vi "Set_DAQmx.vi"(8 "error in (no error)":errorcluster, 11 "Control-Server in":refnum<class "Control-Server.lvclass">) -> (0 "error out":errorcluster, 3 "Control-Server out":refnum<class "Control-Server.lvclass">)   [LabVIEW 2019, in "Control-Server.lvclass"]
uses:
  Control-Server.lvclass
  Config/config_names_def.ctl
  Message/Message.lvclass
  dependecies/ControlsVIs/Clusters-def/Message types.ctl
  Control-Server.lvclass/Control-Server.ctl
  Message/Message.lvclass/Message.ctl
  DAQmxTasks/DAQmxTaskContainer_Emulate/DAQmxTaksContainer_Emulate.lvclass
  C:/Users/elysium/Documents/dev/TRANCON/Classes/DAQmxTasks/DAQmxTaskContainer_General/DAQmxTaksContainer_General.lvclass
  DAQmxTasks/DAQmxTaskContainer/DAQmxTaskContainer.lvclass
  GeneralFunctionality/GeneralFunctionality.lvclass/GeneralFunctionality.ctl
  DAQmxTasks/DAQmxTaskContainer_General/DAQmxTaksContainer_General.lvclass/DAQmxTaksContainer_General.ctl
  Oscilloscope/Oscilloscope.lvclass
  C:/Users/elysium/Documents/dev/TRANCON/Classes/GeneralFunctionality/GeneralFunctionality.lvclass
  Detector/Detector.lvclass
  DAQmxTasks/DAQmxTaskContainer_General/DAQmxTaksContainer_General.lvclass
  Config/Config.lvclass
  GeneralFunctionality/GeneralFunctionality.lvclass
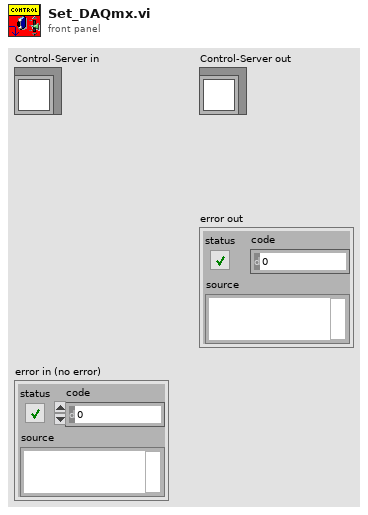
[diagram p1: front panel]
types:
  T1 = typedef "Config.lvclass/config_names_def.ctl" = string
  T2 = typedef "Message types.ctl" = string
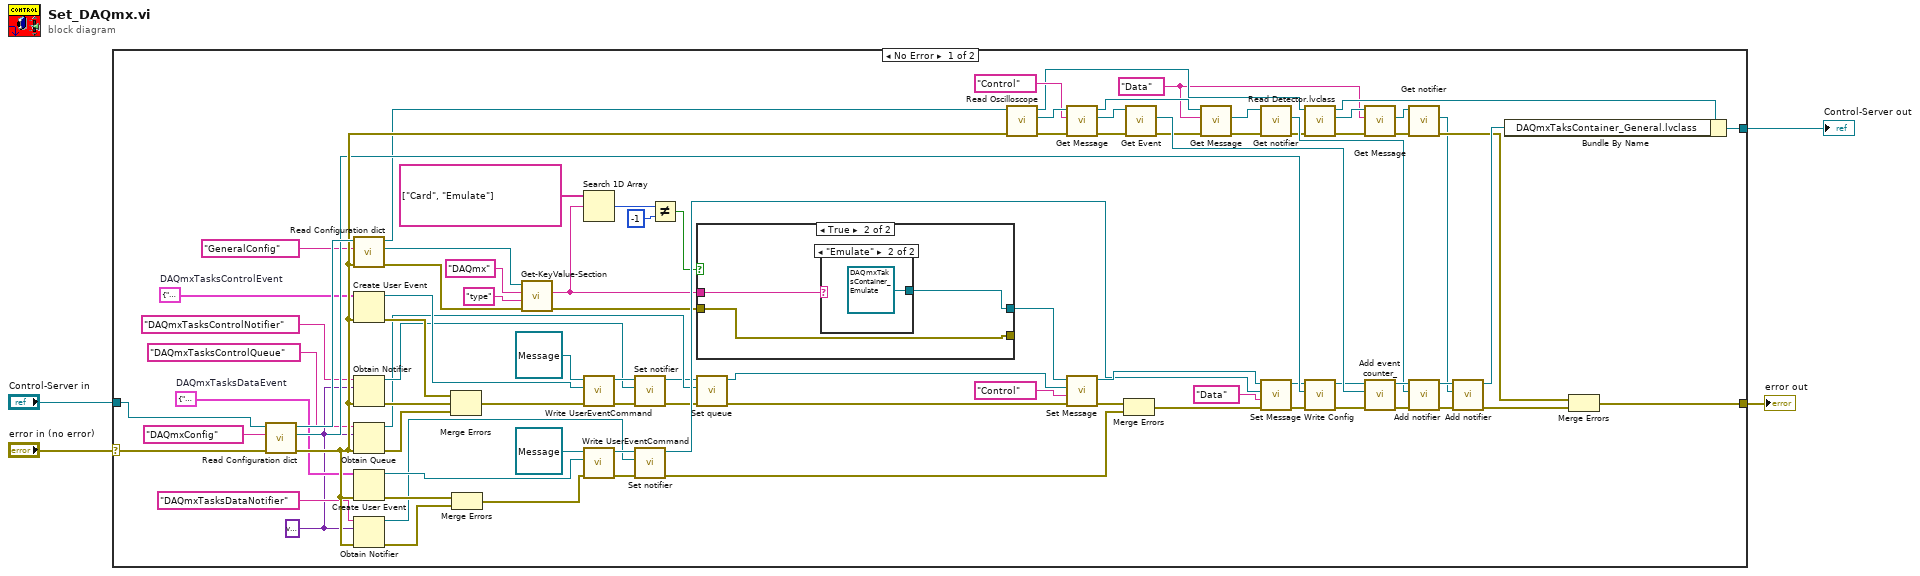
[diagram p0: block diagram]
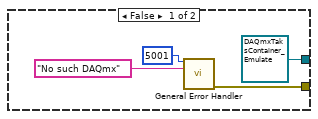
[diagram p2: hidden frame]
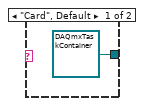
[diagram p3: hidden frame]
diagram:
  n1 = case shown="No Error" "error in (no error)" {
    selector: "error in (no error)" -> [w6 w102]
    tunnel: [w90 w102] -> w4
    tunnel: [w89 w101] -> w3
    tunnel: "Control-Server in" -> [w88 w101]
    frame No Error {
      w24 = T2 "Data" ("Message type")
      w39 = variant
      w71 = cluster{"command":string, "data":variant} {"command"="", "data"=variant}  # DAQmxTasksDataEvent
      w78 = cluster{"command":string, "data":variant} {"command"="", "data"=variant}  # DAQmxTasksControlEvent
      n2 = call "Read Configuration dict.vi"("error in (no error)"=w6, "Config Name"=T1 "DAQmxConfig", "Control in"=w88) -> ("error out"=w85:errorcluster, "Config"=w84:refnum<class "Config.lvclass">, "Control out"=w87:refnum<class "Control-Server.lvclass">)  [unwired: 6 in]
      n3 = call "Read Configuration dict.vi"("error in (no error)"=w85, "Config Name"=T1 "GeneralConfig", "Control in"=w87) -> ("error out"=w19:errorcluster, "Config"=w18:refnum<class "Config.lvclass">, "Control out"=w8:refnum<class "Control-Server.lvclass">)  [unwired: 6 in]
      n4 = Create User Event(user event datatype=w78, error in=w85) -> (user event=w80:refnum<user-event>, error out=w76:errorcluster)
      n5 = Obtain Notifier(name (unnamed)="DAQmxTasksControlNotifier" ("nom (aucun)"), notification data type=w39, error in (no error)=w85) -> (notifier out=w74:refnum<notifier>, error out=w75:errorcluster)  [unwired: 1 in, 1 out]
      n6 = Obtain Queue(name (unnamed)="DAQmxTasksControlQueue", element data type=w39, error in (no error)=w85) -> (queue out=w52:refnum<queue>, error out=w51:errorcluster)  [unwired: 2 in, 1 out]
      n7 = Create User Event(user event datatype=w71, error in=w85) -> (user event=w68:refnum<user-event>, error out=w60:errorcluster)
      n8 = Obtain Notifier(name (unnamed)="DAQmxTasksDataNotifier" ("nom (aucun)"), notification data type=w39, error in (no error)=w85) -> (notifier out=w58:refnum<notifier>, error out=w59:errorcluster)  [unwired: 1 in, 1 out]
      n9 = Merge Errors(w76, w75, w51) -> (w73:errorcluster)
      n10 = Merge Errors(w60, w59) -> (w57:errorcluster)
      n11 = call-dynamic "Get-KeyValue-Section.vi"("error in (no error)"=w19, "Key"="type", "Section"="DAQmx", "Config in"=w18) -> ("error out"=w16:errorcluster, "Value"=w15:string)  [unwired: 5 in, 1 out]
      n12 = Search 1D Array(1D array=string[] ["Card", "Emulate"], element=w15) -> (index of element=w12:i32)  [unwired: 1 in]
      n13 = call "Write UserEventCommand.vi"("error in (no error)"=w73, "UserEventCommand"=w80, "Message en entrée"=refnum<class "Message.lvclass"> refnum ("Message.lvclass")) -> ("error out"=w77:errorcluster, "Message en sortie"=w81:refnum<class "Message.lvclass">)  [unwired: 7 in]
      n14 = call "Write UserEventCommand.vi"("error in (no error)"=w57, "UserEventCommand"=w68, "Message en entrée"=refnum<class "Message.lvclass"> refnum ("Message.lvclass")) -> ("error out"=w66:errorcluster, "Message en sortie"=w67:refnum<class "Message.lvclass">)  [unwired: 7 in]
      n15 = call "Set notifier.vi"("error in (no error)"=w77, "notifier"=w74, "Message en entrée"=w81) -> ("error out"=w50:errorcluster, "Message en sortie"=w48:refnum<class "Message.lvclass">)  [unwired: 7 in]
      n16 = call "Set notifier.vi"("error in (no error)"=w66, "notifier"=w58, "Message en entrée"=w67) -> ("error out"=w55:errorcluster, "Message en sortie"=w61:refnum<class "Message.lvclass">)  [unwired: 7 in]
      n17 = Not Equal?(x=w12, y=-1) -> (x != y?=w14:bool)
      n18 = case shown="True" w14 {
        tunnel: w15 -> [_ w98]
        tunnel: [refnum<class "DAQmxTaksContainer_Emulate.lvclass"> refnum ("DAQmxTaksContainer_Emulate.lvclass") w96] -> w7
        tunnel: w16 -> [_ w97]
        tunnel: [w93 w97] -> _
        frame False {
          n19 = call <vilib>:"General Error Handler.vi"("[error code] (0)"=5001 ("code"), "[error source] (\" \")"="No such DAQmx" ("String to Prepend to source (\"\")")) -> ("error out"=w93:errorcluster)  [unwired: 9 in, 4 out]
        }
        frame True {
          n20 = case shown="\"Emulate\"" w98 {
            tunnel: [refnum<class "DAQmxTaskContainer.lvclass"> refnum ("DAQmxTaskContainer.lvclass") refnum<class "DAQmxTaksContainer_Emulate.lvclass"> refnum ("DAQmxTaksContainer_Emulate.lvclass")] -> w96
            frame "Card", Default {
            }
            frame "Emulate" {
            }
          }
        }
      }
      n21 = call "Set queue.vi"("error in (no error)"=w50, "queue"=w52, "Message in"=w48) -> ("error out"=w49:errorcluster, "Message out"=w47:refnum<class "Message.lvclass">)  [unwired: 7 in]
      n22 = call "Read Oscilloscope.vi"("error in (no error)"=w85, "Control-Server en entrée"=w8) -> ("error out"=w45:errorcluster, "Oscilloscope.lvclass"=w44:refnum<class "Oscilloscope.lvclass">, "Control-Server en sortie"=w27:refnum<class "Control-Server.lvclass">)  [unwired: 7 in]
      n23 = call "Get Message.vi"("error in (no error)"=w45, "Message type"=T2 "Control", "GeneralFunctionality en entrée"=w44) -> ("error out"=w42:errorcluster, "Message.lvclass"=w41:refnum<class "Message.lvclass">, "GeneralFunctionality en sortie"=w33:refnum<class "Oscilloscope.lvclass">)  [unwired: 6 in]
      n24 = call "Set Message.vi"("error in (no error)"=w49, "Message type"=T2 "Control", "Message.lvclass"=w47, "GeneralFunctionality en entrée"=w7) -> ("error out"=w56:errorcluster, "GeneralFunctionality en sortie"=w65:refnum<class "DAQmxTaksContainer_General.lvclass">)  [unwired: 6 in]
      n25 = Merge Errors(w56, w55) -> (w54:errorcluster)
      n26 = call "Get Event.vi"("error in (no error)"=w42, "Message en entrée"=w41) -> ("error out"=w32:errorcluster, "UserEventCommand"=w40:refnum<user-event>)  [unwired: 7 in, 1 out]
      n27 = call "Get Message.vi"("error in (no error)"=w32, "Message type"=w24, "GeneralFunctionality en entrée"=w33) -> ("error out"=w30:errorcluster, "Message.lvclass"=w31:refnum<class "Message.lvclass">)  [unwired: 6 in, 1 out]
      n28 = call "Get notifier.vi"("error in (no error)"=w30, "Message en entrée"=w31) -> ("error out"=w28:errorcluster, "notifier"=w29:refnum<notifier>)  [unwired: 7 in, 1 out]
      n29 = call "Set Message.vi"("error in (no error)"=w54, "Message type"=T2 "Data", "Message.lvclass"=w61, "GeneralFunctionality en entrée"=w65) -> ("error out"=w63:errorcluster, "GeneralFunctionality en sortie"=w64:refnum<class "DAQmxTaksContainer_General.lvclass">)  [unwired: 6 in]
      n30 = call "Read Detector.lvclass.vi"("error in (no error)"=w28, "Control in"=w27) -> ("error out"=w26:errorcluster, "Detector.lvclass"=w25:refnum<class "Detector.lvclass">, "Control out"=w86:refnum<class "Control-Server.lvclass">)  [unwired: 7 in]
      n31 = call "Write Config.vi"("error in (no error)"=w63, "Config.lvclass"=w84, "GeneralFunctionality en entrée"=w64) -> ("error out"=w46:errorcluster, "GeneralFunctionality en sortie"=w5:refnum<class "DAQmxTaksContainer_General.lvclass">)  [unwired: 7 in]
      n32 = call "Get Message.vi"("error in (no error)"=w26, "Message type"=w24, "GeneralFunctionality en entrée"=w25) -> ("error out"=w23:errorcluster, "Message.lvclass"=w20:refnum<class "Message.lvclass">)  [unwired: 6 in, 1 out]
      n33 = call "Add event counter_.vi"("error in (no error)"=w46, "event counter"=w40, "DAQmxTaksContainer_General in"=w5) -> ("error out"=w38:errorcluster, "DAQmxTaksContainer_General out"=w37:refnum<class "DAQmxTaksContainer_General.lvclass">)  [unwired: 7 in]
      n34 = call "Get notifier.vi"("error in (no error)"=w23, "Message en entrée"=w20) -> ("error out"=w22:errorcluster, "notifier"=w21:refnum<notifier>)  [unwired: 7 in, 1 out]
      n35 = call "Add notifier.vi"("error in (no error)"=w38, "notifier"=w29, "DAQmxTaksContainer_General in"=w37) -> ("error out"=w36:errorcluster, "DAQmxTaksContainer_General out"=w35:refnum<class "DAQmxTaksContainer_General.lvclass">)  [unwired: 7 in]
      n36 = call "Add notifier.vi"("error in (no error)"=w36, "notifier"=w21, "DAQmxTaksContainer_General in"=w35) -> ("error out"=w34:errorcluster, "DAQmxTaksContainer_General out"=w83:refnum<class "DAQmxTaksContainer_General.lvclass">)  [unwired: 7 in]
      n37 = Bundle By Name(cluster=w86, "DAQmxTaksContainer_General.lvclass"=w83) -> (w89:refnum<class "Control-Server.lvclass">)
      n38 = Merge Errors(w22, w34) -> (w90:errorcluster)
    }
    frame Error {
    }
  }
  "error out" <- w4
  "Control-Server out" <- w3
